vi "LauncherAngle.vi"() -> ()   [LabVIEW 2012]
uses:
  State_Machine_Enum.ctl
  Robot Global Data.vi
  <vilib>/addons/control/pid/pid.llb/PID (DBL).vi
  <vilib>/addons/control/pid/NI_PID_pid.lvlib
panel:
  in  "PID gains":T1={"proportional gain (Kc)"=1.0, "integral time (Ti, min)"=0.01, "derivative time (Td, min)"=0.0} {"derivative time (Td, min)" format="%.3f"; "integral time (Ti, min)" format="%.3f"; "proportional gain (Kc)" format="%.3f"}
  in  "output range":cluster{"output high":dbl, "output low":dbl}={"output high"=1.0, "output low"=-1.0} {"output low" step=0.1 format="%.2f"; "output high" step=0.1 format="%.2f"}
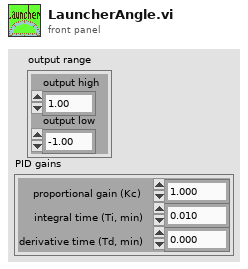
[diagram p1: front panel]
types:
  T1 = cluster{"proportional gain (Kc)":dbl, "integral time (Ti, min)":dbl, "derivative time (Td, min)":dbl}
  T2 = typedef "State_Machine_Enum.ctl" = enum16{"Init", "Idle", "Start", "Do", "Stop"}
  T3 = typedef "WPI_EncoderDevRef.ctl" = cluster{"DevStatus":errorcluster, "EncoderIndex":T4, "CounterIndex":T5, "DistancePerCount":dbl, "Decoding Type":T6}
  T4 = typedef "FPGA_EncoderIdx.ctl" = enum8{"Enc 0", "Enc 1", "Enc 2", "Enc 3", "Invalid"}
  T5 = typedef "FPGA_CounterCtrSystemIndex.ctl" = enum8{"Ctr 0", "Ctr 1", "Ctr 2", "Ctr 3", "Ctr 4", "Ctr 5", "Ctr 6", "Ctr 7", "Invalid"}
  T6 = typedef "WPI_EncoderType.ctl" = enum16{"1x", "2x", "4x"}
  T7 = typedef "WPI_MotorControlDeviceRef.ctl" = cluster{"DeviceStatus":errorcluster, "Type":enum16{"PWM", "CAN"}, "PWM":cluster{"Digital Module":T8, "PWM Channel":T9, "DeadBand":T10}, "CAN":cluster{"Device Number":u8, "Control Mode":T11, "Semaphore":T12, "Max Vout":dbl}, "Invert":bool, "TransformRef":T13, "InvTransformRef":T13}
  T8 = typedef "FPGA_TypedefDigitalModule.ctl" = enum16{"Digital Module 1", "Digital Module 2"}
  T9 = typedef "FPGA_DIOPWMChannel.ctl" = enum8{"PWM 1", "PWM 2", "PWM 3", "PWM 4", "PWM 5", "PWM 6", "PWM 7", "PWM 8", "PWM 9", "PWM 10", "Invalid"}
  T10 = typedef "WPI_PWMDeadband.ctl" = cluster{"Name":string, "maxPositivePwm":i32, "minPositivePwm":i32, "centerPwm":i32, "maxNegativePwm":i32, "minNegativePwm":i32, "angularRange":u16}
  T11 = typedef "WPI_CANJaguar_ControlMode.ctl" = enum8{"Percent VBus", "Current", "Speed", "Position", "Voltage"}
  T12 = typedef "Semaphore RefNum" = refnum<k1>
  T13 = typedef "WPI_PWMTransform_ConPane.ctl" = refnum<vi>
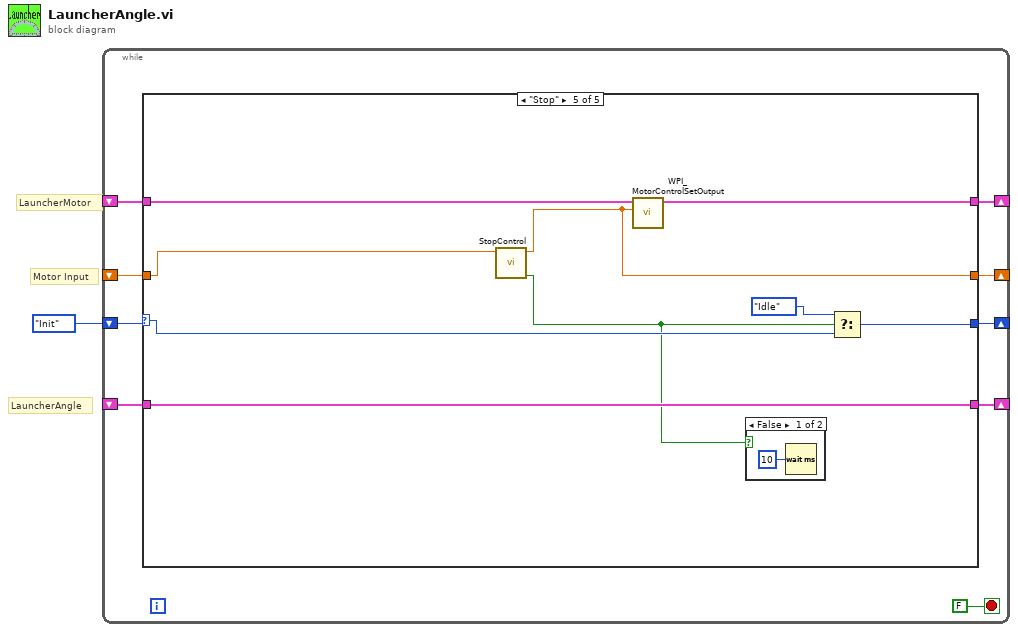
[diagram p0: block diagram]
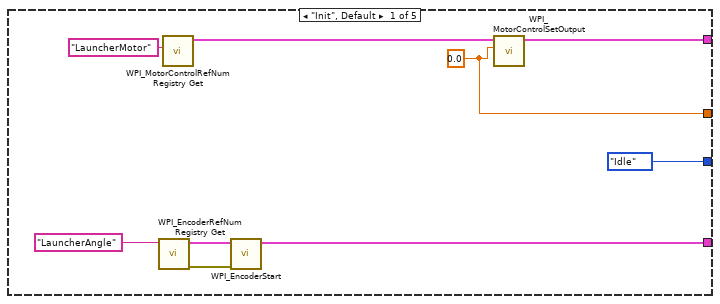
[diagram p2: hidden frame]
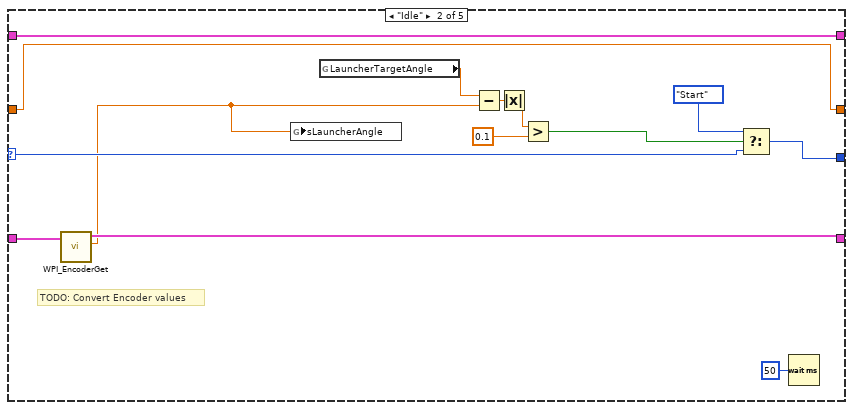
[diagram p3: hidden frame]
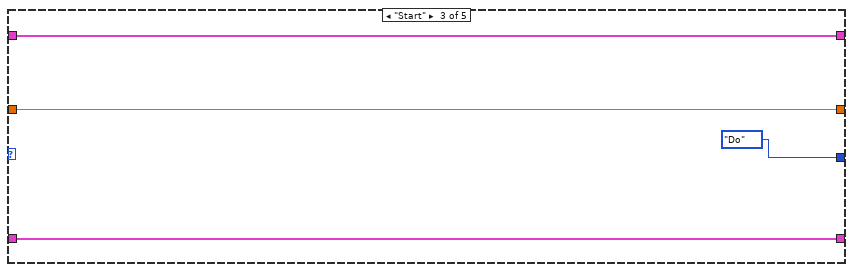
[diagram p4: hidden frame]
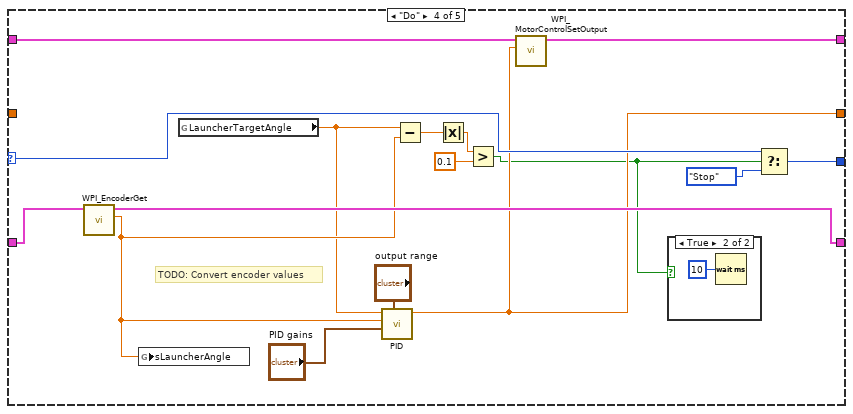
[diagram p5: hidden frame]
diagram:
  # "LauncherAngle"
  # "Motor Input"
  # "LauncherMotor"
  n1 = while {
    shift-right: [w8] -> _
    shift-left: State_Machine_Enum."Init" ("State") -> [w9]
    shift-right: [w7] -> _
    shift-left: _ -> [w6]
    shift-right: [w5] -> _
    shift-left: _ -> [w4]
    shift-right: [w3] -> _
    shift-left: _ -> [w2]
    stop <- FALSE stop-if-true
    n2 = case shown="\"Stop\"" w9 {
      selector: w9 -> [_ w26 _ w43 w57]
      tunnel: [State_Machine_Enum."Idle" ("State") w28 State_Machine_Enum."Do" ("State") w42 w58] -> w8
      tunnel: [w13 w31 w36 w50 w63] -> w7
      tunnel: w6 -> [_ w32 w36 w51 w63]
      tunnel: [w14 w21 w35 w48 w60] -> w5
      tunnel: w4 -> [_ w21 w35 w49 w61]
      tunnel: [w12 w20 w34 w41 w56] -> w3
      tunnel: w2 -> [_ w20 w34 _ w62]
      frame "Init", Default {
        w12 = 0.0 ("Output")
        n3 = call <vilib>:"WPI_EncoderRefNum Registry Get.vi"("refnum name"="LauncherAngle") -> ("error out"=w11:errorcluster, "EncoderDevRef"=w17:T3)  [unwired: 9 in]
        n4 = call <vilib>:"WPI_MotorControlRefNum Registry Get.vi"("refnum name"="LauncherMotor") -> ("MotorControlDevRef"=w15:T7)  [unwired: 9 in, 1 out]
        n5 = call <vilib>:"WPI_EncoderStart.vi"("error in (no error)"=w11, "EncoderDevRef"=w17) -> ("EncoderDevRef"=w13:T3)  [unwired: 8 in, 1 out]
        n6 = call <vilib>:"WPI_MotorControlSetOutput.vi"("Output"=w12, "MotorControlDevRef"=w15) -> ("MotorControlDevRef"=w14:T7)  [unwired: 7 in, 2 out]
      }
      frame "Idle" {
        # "TODO: Convert Encoder values"
        n7 = call <vilib>:"WPI_EncoderGet.vi"("EncoderDevRef"=w32) -> ("Distance"=w22:dbl, "EncoderDevRef"=w31:T3)  [unwired: 5 in, 4 out]
        n8 = global write "Robot Global Data.vi" "sLauncherAngle"(w22) -> ()
        n9 = global read "Robot Global Data.vi" "LauncherTargetAngle"() -> (w33:dbl)
        n10 = Subtract(x=w33, y=w22) -> (x-y=w30:dbl)
        n11 = Absolute Value(x=w30) -> (abs(x)=w25:dbl)
        n12 = Greater?(x=w25, y=0.1) -> (0:w27:bool)
        n13 = Select(t=State_Machine_Enum."Start" ("State"), s=w27, f=w26) -> (s? t:f=w28:T2)
        n14 = Wait (ms)(milliseconds to wait=u32 50) -> ()  [unwired: 1 out]
      }
      frame "Start" {
      }
      frame "Do" {
        # "TODO: Convert encoder values"
        n15 = call <vilib>:"WPI_EncoderGet.vi"("EncoderDevRef"=w51) -> ("Distance"=w40:dbl, "EncoderDevRef"=w50:T3)  [unwired: 5 in, 4 out]
        n16 = global write "Robot Global Data.vi" "sLauncherAngle"(w40) -> ()
        n17 = global read "Robot Global Data.vi" "LauncherTargetAngle"() -> (w39:dbl)
        n18 = call-poly <vilib>:"PID.vi"("output range"="output range", "PID gains"="PID gains", "process variable"=w40, "setpoint"=w39) -> ("output"=w41:dbl)  [unwired: 6 in, 1 out]
        n19 = Subtract(x=w39, y=w40) -> (x-y=w47:dbl)
        n20 = Absolute Value(x=w47) -> (abs(x)=w46:dbl)
        n21 = Greater?(x=w46, y=0.1) -> (0:w38:bool)
        n22 = call <vilib>:"WPI_MotorControlSetOutput.vi"("Output"=w41, "MotorControlDevRef"=w49) -> ("MotorControlDevRef"=w48:T7)  [unwired: 7 in, 2 out]
        n23 = case shown="True" w38 {
          frame False {
          }
          frame True {
            n24 = Wait (ms)(milliseconds to wait=u32 10) -> ()  [unwired: 1 out]
          }
        }
        n25 = Select(t=w43, s=w38, f=State_Machine_Enum."Stop" ("State")) -> (s? t:f=w42:T2)
      }
      frame "Stop" {
        n26 = call "StopControl.vi"("Motor Value"=w62) -> ("Done Stopping"=w55:bool, "New Motor Value"=w56:dbl)  [unwired: 9 in]
        n27 = call <vilib>:"WPI_MotorControlSetOutput.vi"("Output"=w56, "MotorControlDevRef"=w61) -> ("MotorControlDevRef"=w60:T7)  [unwired: 7 in, 2 out]
        n28 = case shown="False" w55 {
          frame False {
            n29 = Wait (ms)(milliseconds to wait=u32 10) -> ()  [unwired: 1 out]
          }
          frame True {
          }
        }
        n30 = Select(t=State_Machine_Enum."Idle" ("State"), s=w55, f=w57) -> (s? t:f=w58:T2)
      }
    }
  }
